vi "Power_spectrum_TF.vi"(5 "Spectrum input array":dbl[](array[numeric]) format="%.2f", 7 "Smoothing":enum16{"Linear", "Logarithmic"}(ring), 8 "Cluster 1":T2={"Colour"=0, "Inst type"=enum."Pitot-static tube", "Inst name"="Manometer voltage", "Symbol"="U", "Code name"="", "Extra Info"="U", "Inst Array"=enum."PWA", "Index"=0, "Voltage Index"=0, "Extra Titles"=[], "Extra Values"=[], "Eng Values"=[], "Time (ms)"=[], "TT / Voltage"=[], "U"=0.0, "u^2"=0.0, "u^3"=0.0, "u^4"=0.0, "Skew_u"=0.0, "Kurt_u"=0.0, "Mean % Err"=0.0, "% u'/U"=0.0} {"Skew_u" format="%.2f"; "% u'/U" format="%.2f"; "Mean % Err" format="%.2f"; "Kurt_u" format="%.2f"; "u^4" format="%.2f"; "u^3" format="%.2f"; "U" format="%.2f"; "u^2" format="%.2f"}) -> (0 "Spectrum output array":dbl[](array[numeric]) format="%.2f", 2 "XY Graph":cluster{dbl[], dbl[]}(graph), 3 "XY Plot Cluster":T1)   [LabVIEW 2011]
uses:
  Controls/Analysis_info_cluster.ctl
  Controls/Inst_type.ctl
  Controls/Instrument_Array.ctl
  Controls/XY_Plot_Cluster.ctl
  Globals/Meas_global.vi
  <vilib>/Analysis/baseanly.llb/Scale 1D.vi
  <vilib>/gmath/NI_Gmath.lvlib
  <vilib>/Analysis/NI_AALBase.lvlib
panel:
  out "XY Graph 2":cluster{dbl[], dbl[]}(graph)
  in  "method":i32(ring) items=["nearest", "linear", "spline", "cubic Hermite", "Lagrange"]
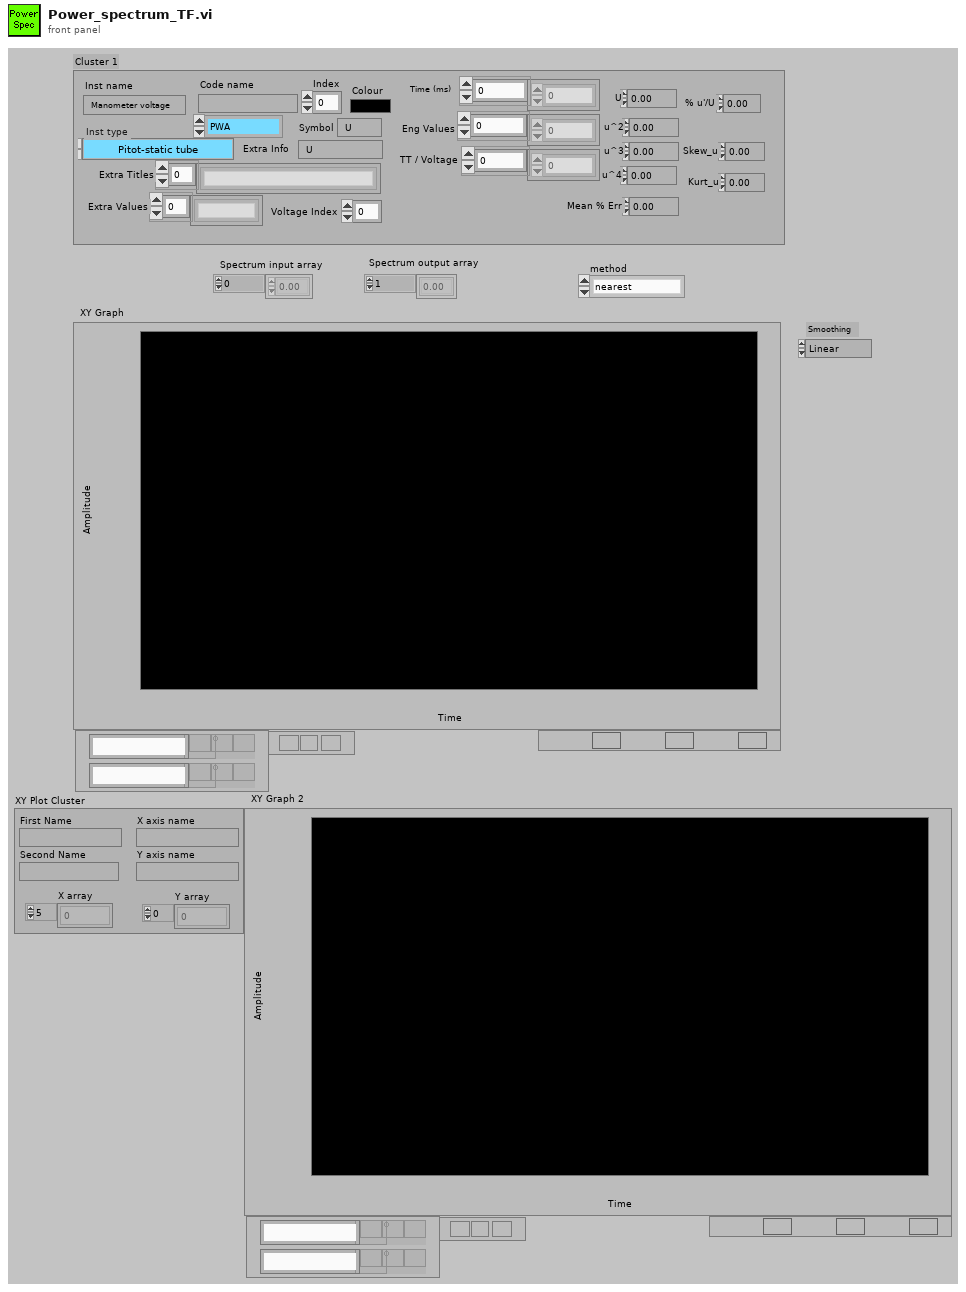
[diagram p1: front panel]
types:
  T1 = typedef "XY_Plot_Cluster.ctl" = cluster{"First Name":string, "Second Name":string, "X axis name":string, "Y axis name":string, "X array":dbl[], "Y array":dbl[]}
  T2 = typedef "Analysis_info_cluster.ctl" = cluster{"Colour":u32, "Inst type":T3, "Inst name":string, "Symbol":string, "Code name":string, "Extra Info":string, "Inst Array":T4, "Index":i32, "Voltage Index":i32, "Extra Titles":string[], "Extra Values":string[], "Eng Values":dbl[], "Time (ms)":dbl[], "TT / Voltage":dbl[], "U":dbl, "u^2":dbl, "u^3":dbl, "u^4":dbl, "Skew_u":dbl, "Kurt_u":dbl, "Mean % Err":dbl, "% u'/U":dbl}
  T3 = typedef "Inst_type.ctl" = enum16{"Propeller anemometer", "Raw voltage", "Pressure Transducer", "Pitot-static tube", "Preston tube", "Hot wire", "Cross wire 1", "Cross wire 2", "Generic Linear", "Generic Polynomial", "Generic BackPoly", "Fast FID", "Thermocouple", "Cold wire", "Pulsed Wire", "LDA Vel", "LDA Tran time", "LDA Arr time"}
  T4 = typedef "Instrument_Array.ctl" = enum16{"PWA", "LDA", "Analogue"}
  T5 = cluster{"X array Out":dbl[], "Y array Out":dbl[]}
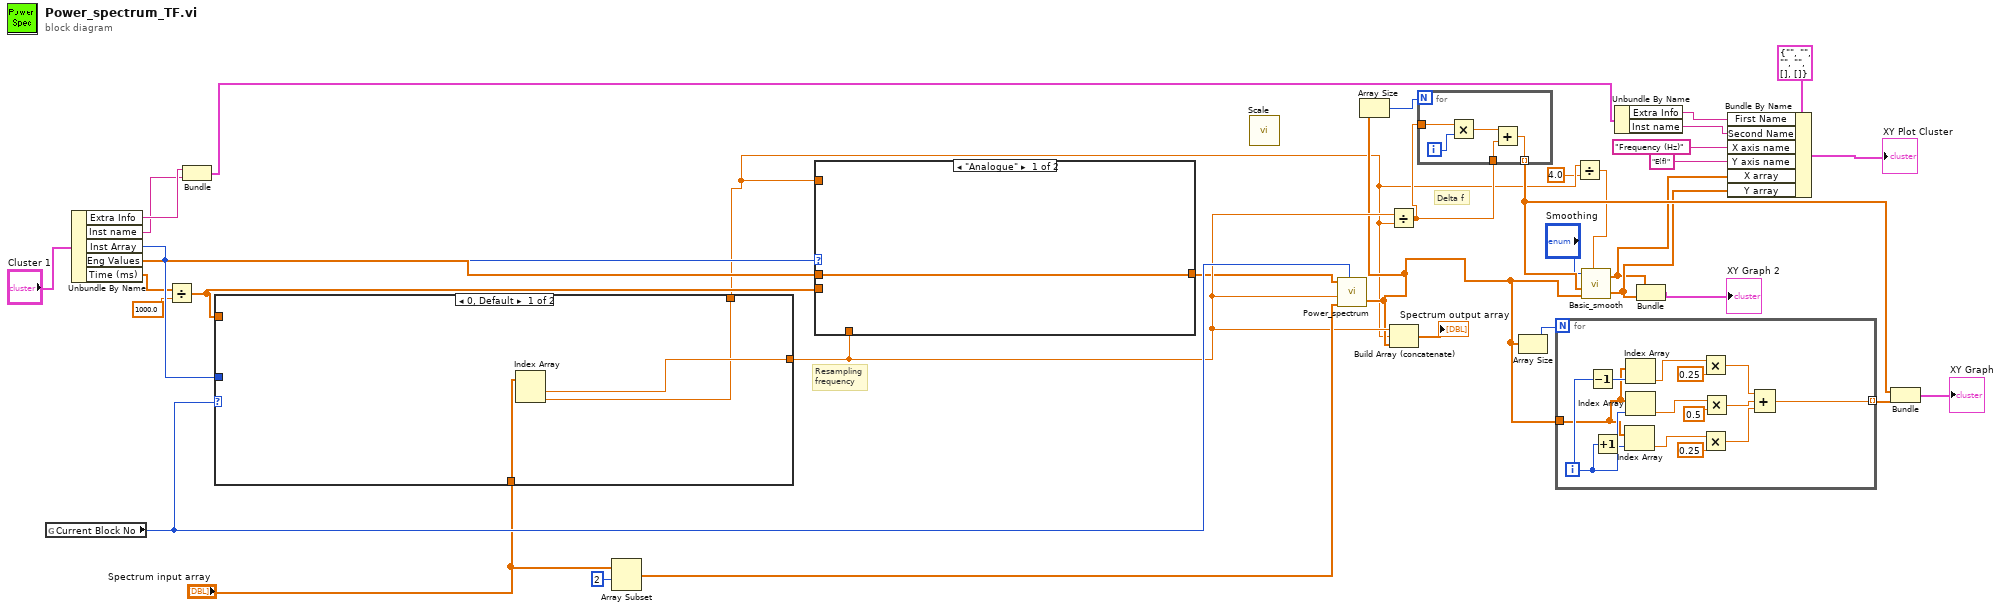
[diagram p0: block diagram]
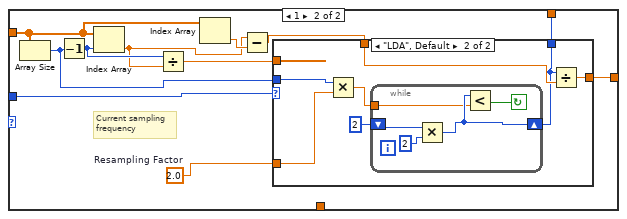
[diagram p2: hidden frame]
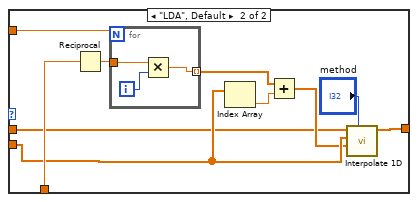
[diagram p4: hidden frame]
diagram:
  # "Resampling\nfrequency"
  # "Delta f"
  n1 = global read "Meas_global.vi" "Current Block No"() -> (w34:i32)
  n2 = Unbundle By Name("Cluster 1") -> ("Extra Info"=w12:string, "Inst name"=w10:string, "Inst Array"=w29:T4, "Eng Values"=w35:dbl[], "Time (ms)"=w26:dbl[])
  n3 = Divide(x=w26, y=1000.0) -> (x/y=w25:dbl[])
  n4 = Bundle("Extra Info"=w12, "Inst name"=w10) -> (w11:cluster{"Extra Info":string, "Inst name":string})  [unwired: 1 in]
  n5 = case shown="0, Default" w34 {
    tunnel: w25 -> [_ w43]
    tunnel: [w38 w48] -> w28
    tunnel: "Spectrum input array" -> [w39 _]
    tunnel: w29 -> [_ w49]
    tunnel: [w37 w46] -> w16
    frame 0, Default {
      n6 = Index Array(array=w39) -> (element #1=w38:dbl, element #2=w37:dbl)  [unwired: 2 in]
    }
    frame 1 {
      w44 = 2.0  # Resampling Factor
      # "Current sampling\nfrequency"
      n7 = Array Size(array=w43) -> (size(s)=w45:i32)
      n8 = Decrement(x=w45) -> (x-1=w47:i32)
      n9 = Index Array(array=w43, index=w47) -> (element=w40:dbl)
      n10 = Divide(x=w47, y=w40) -> (x/y=w50:dbl)
      n11 = Index Array(array=w43) -> (element=w42:dbl)  [unwired: 1 in]
      n12 = Subtract(x=w40, y=w42) -> (x-y=w41:dbl)
      n13 = case shown="\"LDA\", Default" w49 {
        tunnel: w50 -> [w52 _]
        tunnel: w41 -> [_ w59]
        tunnel: [w52 w58] -> w48
        tunnel: w45 -> [w51 w56]
        tunnel: [w51 w55] -> w46
        tunnel: w44 -> [_ w54]
        frame "Analogue" {
        }
        frame "LDA", Default {
          n14 = Multiply(x=w56, y=w54) -> (x*y=w57:dbl)
          n15 = while {
            shift-right: [w62] -> w55
            shift-left: 2 -> [w64]
            tunnel: w57 -> [w60]
            stop <- w61 continue-if-true
            n16 = Multiply(x=w64, y=2) -> (x*y=w62:i32)
            n17 = Less?(x=w62, y=w60) -> (x < y?=w61:bool)
          }
          n18 = Divide(x=w55, y=w59) -> (x/y=w58:dbl)
        }
      }
    }
  }
  n19 = Array Subset(array="Spectrum input array", index=2) -> (w31:dbl[])  [unwired: 1 in]
  n20 = case shown="\"Analogue\"" w29 {
    tunnel: w35 -> [w65 w66]
    tunnel: w25 -> [_ w70]
    tunnel: [w65 w74] -> w1
    tunnel: w16 -> [_ w73]
    tunnel: w28 -> [_ w71]
    frame "Analogue" {
    }
    frame "LDA", Default {
      n21 = Reciprocal(x=w71) -> (1/x=w72:dbl)
      n22 = for {
        N: w73 -> [_]
        tunnel: w72 -> [w78]
        tunnel: [w76] -> w68 mode=indexing
        i -> [w77]
        n23 = Multiply(x=w78, y=w77) -> (x*y=w76:dbl)
      }
      n24 = Index Array(array=w70) -> (element=w69:dbl)  [unwired: 1 in]
      n25 = Add(x=w68, y=w69) -> (x+y=w67:dbl[])
      n26 = call <vilib>:"Interpolate 1D.vi"("method"="method", "xi"=w67, "X"=w70, "Y"=w66) -> ("yi"=w74:dbl[])  [unwired: 2 in, 5 out]
    }
  }
  n27 = call-poly <vilib>:"Scale.vi"() -> ()  [unwired: 1 in, 4 out]
  n28 = call "Power_spectrum.vi"("U"=w1, "Sampling frequency"=w28, "Spectrum input array"=w31, "Block No"=w34) -> ("Spectrum output array"=w18:dbl[])  [unwired: 2 in]
  n29 = Array Size(array=w18) -> (size(s)=w23:i32)
  n30 = Divide(x=w28, y=w16) -> (x/y=w24:dbl)
  n31 = Build Array (concatenate)(w28, w16, w18) -> (→"Spectrum output array":dbl[])
  n32 = for {
    N: w23 -> [_]
    tunnel: w24 -> [w83]
    tunnel: w24 -> [w80]
    tunnel: [w79] -> w19 mode=indexing
    i -> [w82]
    n33 = Multiply(x=w83, y=w82) -> (x*y=w81:dbl)
    n34 = Add(x=w81, y=w80) -> (x+y=w79:dbl)
  }
  n35 = Array Size(array=w18) -> (size(s)=w21:i32)
  n36 = for {
    N: w21 -> [_]
    tunnel: w18 -> [w89]
    tunnel: [w84] -> w22 mode=indexing
    i -> [w96]
    n37 = Decrement(x=w96) -> (x-1=w97:i32)
    n38 = Increment(x=w96) -> (x+1=w95:i32)
    n39 = Index Array(array=w89, index=w95) -> (element=w90:dbl)
    n40 = Index Array(array=w89, index=w97) -> (element=w93:dbl)
    n41 = Index Array(array=w89, index=w96) -> (element=w88:dbl)
    n42 = Multiply(x=w93, y=0.25) -> (x*y=w87:dbl)
    n43 = Multiply(x=w90, y=0.25) -> (x*y=w85:dbl)
    n44 = Multiply(x=w88, y=0.5) -> (x*y=w86:dbl)
    n45 = Compound Arithmetic op=ADD(w87, w86, w85) -> (w84:dbl)
  }
  n46 = Divide(x=w16, y=4.0) -> (x/y=w14:dbl)
  n47 = call "Basic_smooth.vi"("Smoothing"="Smoothing", "X array in"=w19, "Y array in"=w18, "No of estimates output"=w14) -> ("X array Out"=w5:dbl[], "Y array Out"=w6:dbl[])  [unwired: 1 out]
  n48 = Unbundle By Name(w11) -> ("Extra Info"=w8:string, "Inst name"=w7:string)
  n49 = Bundle("X array Out"=w5, "Y array Out"=w6) -> (→"XY Graph 2":T5)  [unwired: 1 in]
  n50 = Bundle By Name(cluster=T1 {"First Name"="", "Second Name"="", "X axis name"="", "Y axis name"="", "X array"=[], "Y array"=[]} ("output cluster"), "First Name"=w8, "Second Name"=w7, "X axis name"="Frequency (Hz)", "Y axis name"="E(f)", "X array"=w5, "Y array"=w6) -> (→"XY Plot Cluster":T1)
  n51 = Bundle(w19, w22) -> (→"XY Graph":cluster{dbl[], dbl[]})  [unwired: 1 in]
